vi "RANGE Grab Bank Data.vi"(0 "DAQ Data In in":T4, 1 "Meter Number":T10, 2 "Tot.Flow (Liters) Bank 2":dbl, 3 "Use Mass Flow Unit Converter?":bool, 5 "Meter Select":T3, 7 "Tot.Flow (Liters) Bank 1":dbl, 9 "Meter Select 2":T1, 11 "error in (no error)":errorcluster, 12 "Meter Select 3":T2, 13 "Tot.Flow (Liters) Bank 3":dbl) -> (4 "DAQ Data In out":T4, 15 "error out":errorcluster)   [LabVIEW 2018]
uses:
  Type Definitions/RANGE DAQ Data Four Meters.ctl
  Type Definitions/RANGE DAQ Data.ctl
  Drivers/Omega FMA-1600A Series Gas Flow Meter/Type Definitions/FMA1600A Gas Type.ctl
  Drivers/Omega FMA-1600A Series Gas Flow Meter/Type Definitions/FMA1600A Units String.ctl
  Type Definitions/RANGE GAS Data.ctl
  Type Definitions/RANGE Panel Data.ctl
  Type Definitions/Range Meter Bank.ctl
  Type Definitions/RANGE Meter Selector 1-2.ctl
  Type Definitions/RANGE Meter Selector 5-6.ctl
  Type Definitions/RANGE Meter Selector 3-4.ctl
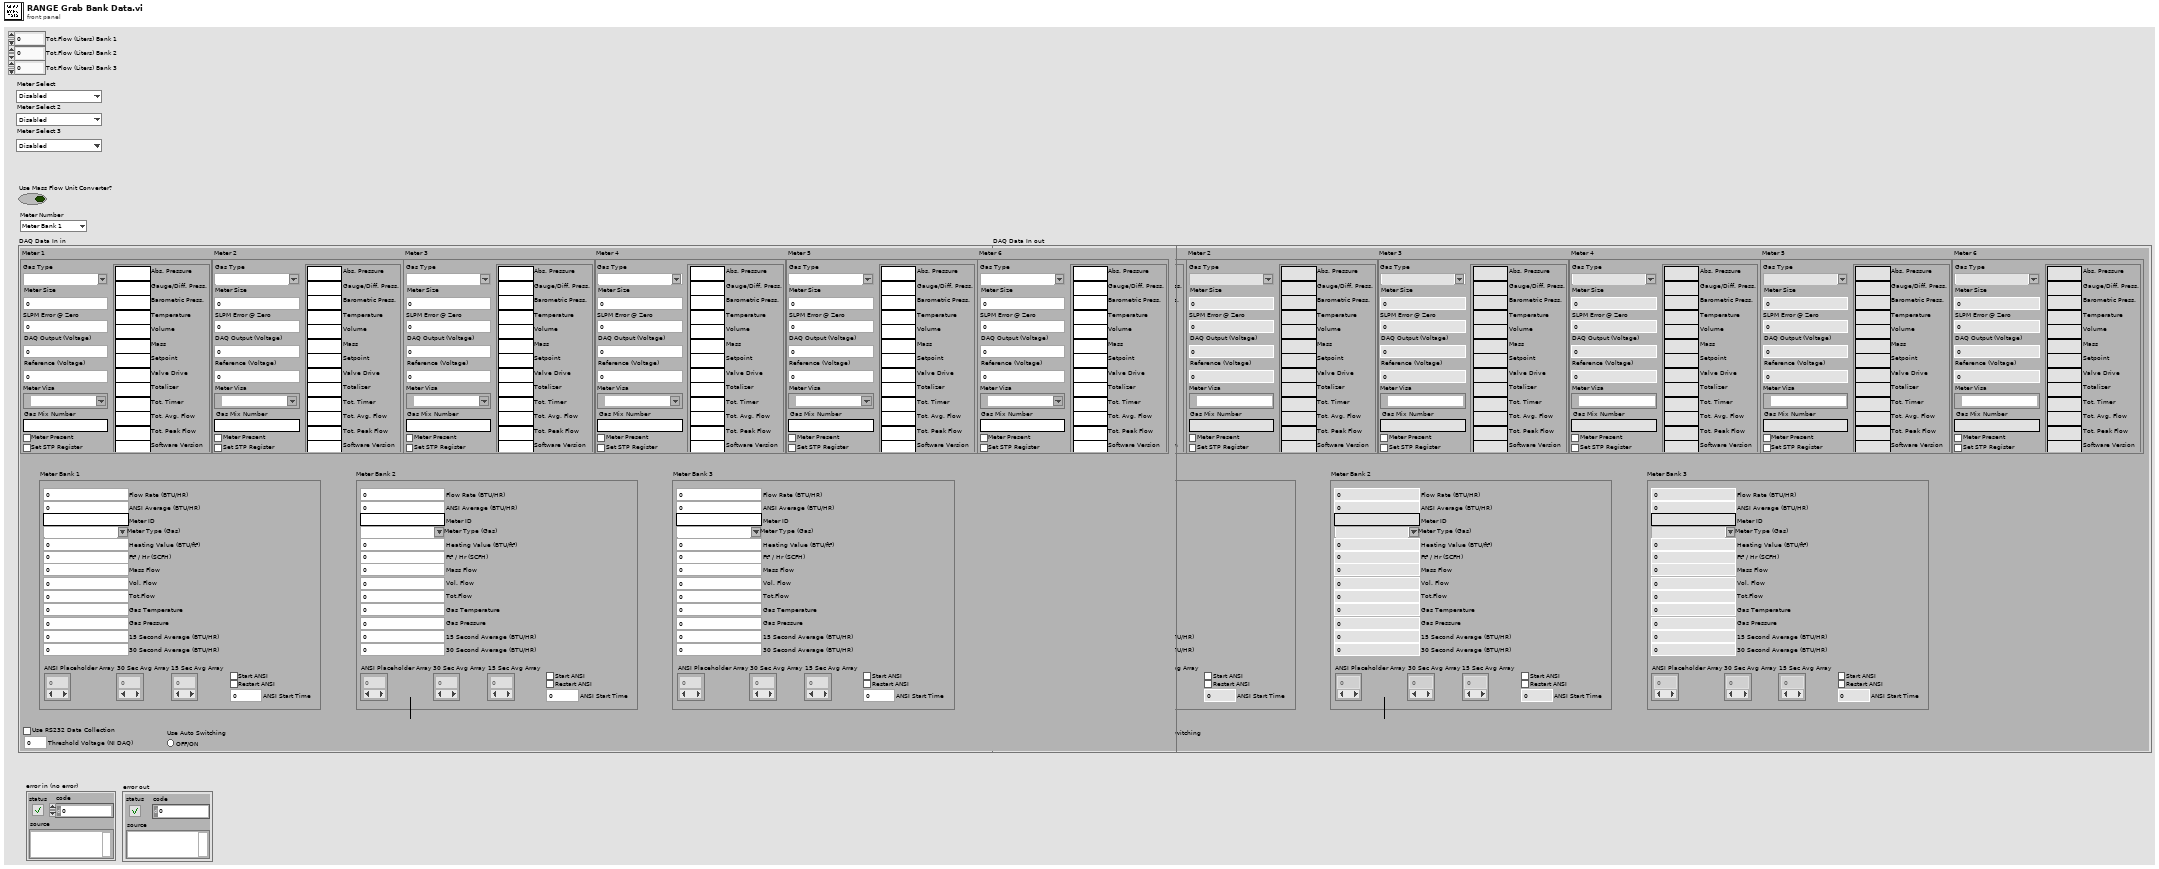
[diagram p1: front panel]
types:
  T1 = typedef "RANGE Meter Selector 3-4.ctl" = enum16{"Disabled", "Meter 3", "Meter 4", "Auto"}
  T2 = typedef "RANGE Meter Selector 5-6.ctl" = enum16{"Disabled", "Meter 5", "Meter 6", "Auto"}
  T3 = typedef "RANGE Meter Selector 1-2.ctl" = enum16{"Disabled", "Meter 1", "Meter 2", "Auto"}
  T4 = typedef "RANGE DAQ Data Four Meters.ctl" = cluster{"Meter 1":T5, "Meter 2":T5, "Meter 3":T5, "Meter 4":T5, "Meter 5":T5, "Meter 6":T5, "Meter Bank 1":T8, "Meter Bank 2":T8, "Meter Bank 3":T8, "Threshold Voltage (NI DAQ)":dbl, "Use RS232 Data Collection":bool, "Use Auto Switching":bool}
  T5 = typedef "RANGE DAQ Data.ctl" = cluster{"Meter Size":dbl, "DAQ Output (Voltage)":dbl, "Reference (Voltage)":dbl, "Meter Present":bool, "Meter Visa":refnum<visa-resource-name>, "Gas Type":T6, "SLPM Error @ Zero":dbl, "Gas Mix Number":string, "Set STP Register":bool, "Measurement Units":T7}
  T6 = typedef "FMA1600A Gas Type.ctl" = string
  T7 = typedef "FMA1600A Units String.ctl" = cluster{"Abs. Pressure":string, "Gauge/Diff. Press.":string, "Barometric Press.":string, "Temperature":string, "Volume":string, "Mass":string, "Setpoint":string, "Valve Drive":string, "Totalizer":string, "Tot. Timer":string, "Tot. Avg. Flow":string, "Tot. Peak Flow":string, "Software Version":string}
  T8 = typedef "RANGE GAS Data.ctl" = cluster{"Flow Rate (BTU/HR)":dbl, "ANSI Placeholder Array":dbl[], "15 Sec Avg Array":dbl[], "30 Sec Avg Array ":dbl[], "ANSI Average (BTU/HR)":dbl, "Panel Data":T9, "Start ANSI":bool, "ANSI Start Time":dbl, "Restart ANSI":bool, "Meter ID":string}
  T9 = typedef "RANGE Panel Data.ctl" = cluster{"Meter Type (Gas)":T6, "Heating Value (BTU/ft³)":dbl, "Ft³ / Hr (SCFH)":dbl, "15 Second Average (BTU/HR)":dbl, "30 Second Average (BTU/HR)":dbl, "Mass Flow":dbl, "Vol. Flow":dbl, "Gas Temperature":dbl, "Gas Pressure":dbl, "Tot.Flow":dbl}
  T10 = typedef "Range Meter Bank.ctl" = enum16{"Meter Bank 1", "Meter Bank 2", "Meter Bank 3"}
  T11 = typedef "FMA1600A Data.ctl" = cluster{"Pressure (PSIA)":dbl, "Temperature (°F)":dbl, "Vol. Flow (LPM)":dbl, "Mass Flow (SLPM)":dbl, "Gas Type":string, "Tot. Flow (Liters)":dbl, "Meter ID":string}
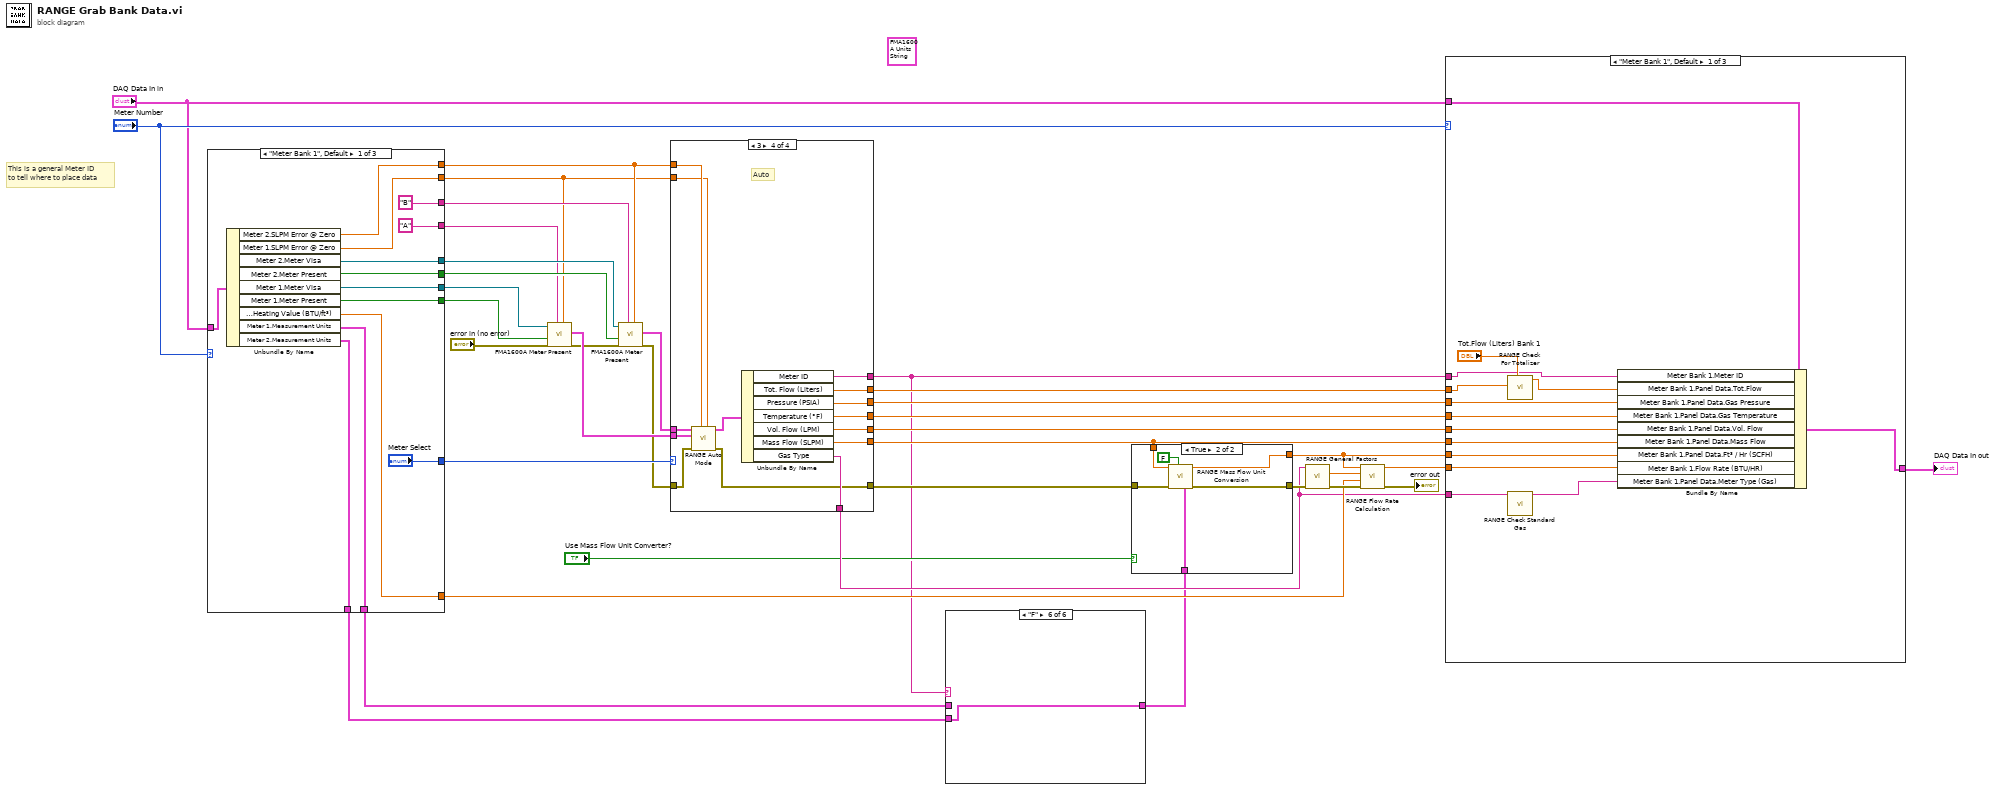
[diagram p0: block diagram]
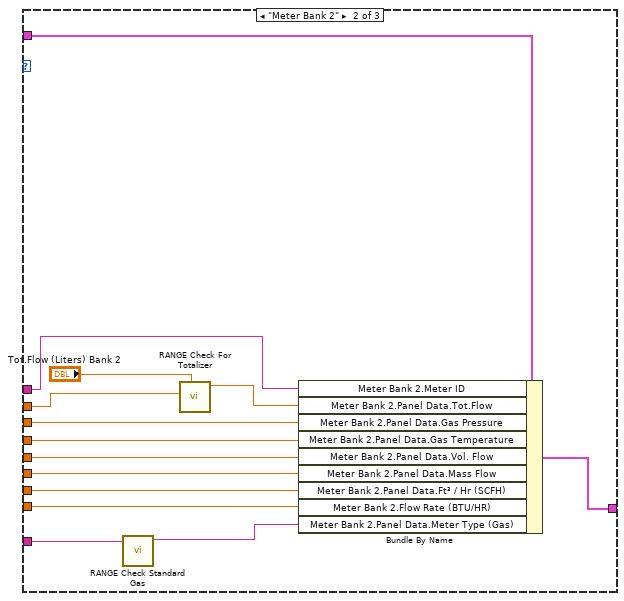
[diagram p8: hidden frame]
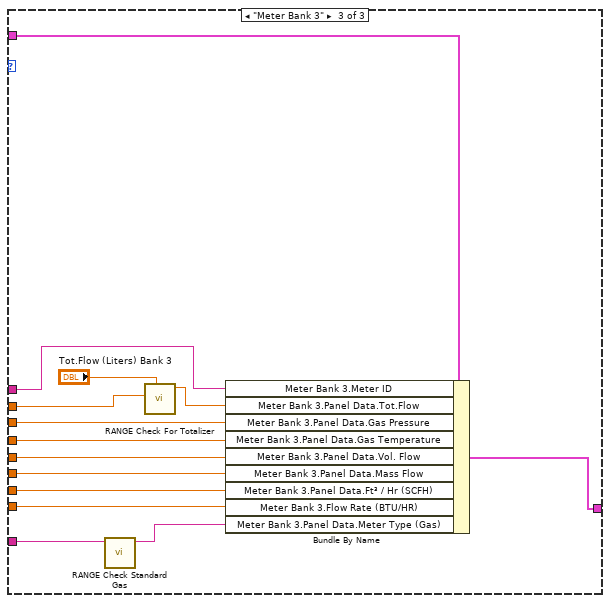
[diagram p9: hidden frame]
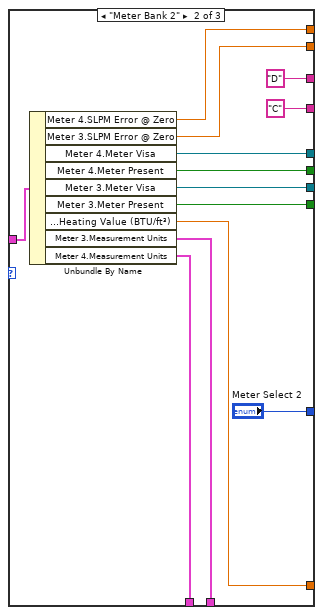
[diagram p10: hidden frame]
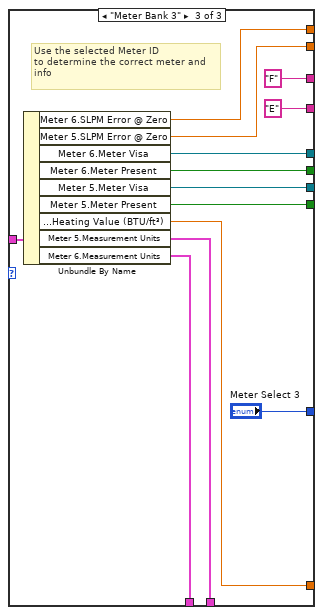
[diagram p11: hidden frame]
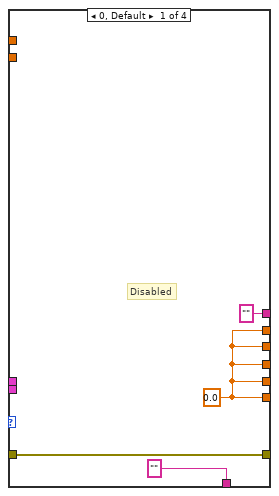
[diagram p12: hidden frame]
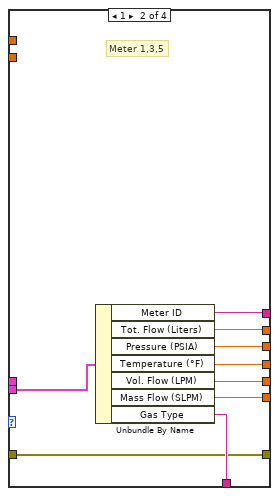
[diagram p13: hidden frame]
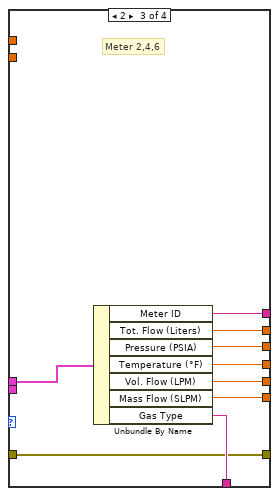
[diagram p14: hidden frame]
diagram:
  (unwired) T7 {"Abs. Pressure"="", "Gauge/Diff. Press."="", "Barometric Press."="", "Temperature"="", "Volume"="", "Mass"="", "Setpoint"="", "Valve Drive"="", "Totalizer"="", "Tot. Timer"="", "Tot. Avg. Flow"="", "Tot. Peak Flow"="", "Software Version"=""} ("Measurement Units")
  # "This is a general Meter ID\nto tell where to place data"
  n1 = case shown="\"Meter Bank 1\", Default" "Meter Number" {
    tunnel: ["A" ("Unit ID") "C" ("Unit ID") "E" ("Unit ID")] -> w22
    tunnel: [w48 w58 w71] -> w5
    tunnel: ["B" ("Unit ID") "D" ("Unit ID") "F" ("Unit ID")] -> w21
    tunnel: "DAQ Data In in" -> [w46 w60 w73]
    tunnel: ["Meter Select" "Meter Select 2" "Meter Select 3"] -> w34
    tunnel: [w45 w59 w72] -> w25
    tunnel: [w44 w57 w70] -> w27
    tunnel: [w43 w56 w69] -> w24
    tunnel: [w42 w55 w67] -> w7
    tunnel: [w41 w54 w68] -> w6
    tunnel: [w40 w53 w66] -> w13
    tunnel: [w38 w50 w63] -> w2
    tunnel: [w37 w51 w64] -> w3
    frame "Meter Bank 1", Default {
      n2 = Unbundle By Name(w46) -> ("Meter 2.SLPM Error @ Zero"=w42:dbl, "Meter 1.SLPM Error @ Zero"=w41:dbl, "Meter 2.Meter Visa"=w45:refnum<visa-resource-name>, "Meter 2.Meter Present"=w43:bool, "Meter 1.Meter Visa"=w48:refnum<visa-resource-name>, "Meter 1.Meter Present"=w44:bool, "Meter Bank 1.Panel Data.Heating Value (BTU/ft³)"=w40:dbl, "Meter 1.Measurement Units"=w37:T7, "Meter 2.Measurement Units"=w38:T7)
    }
    frame "Meter Bank 2" {
      n3 = Unbundle By Name(w60) -> ("Meter 4.SLPM Error @ Zero"=w55:dbl, "Meter 3.SLPM Error @ Zero"=w54:dbl, "Meter 4.Meter Visa"=w59:refnum<visa-resource-name>, "Meter 4.Meter Present"=w56:bool, "Meter 3.Meter Visa"=w58:refnum<visa-resource-name>, "Meter 3.Meter Present"=w57:bool, "Meter Bank 2.Panel Data.Heating Value (BTU/ft³)"=w53:dbl, "Meter 3.Measurement Units"=w51:T7, "Meter 4.Measurement Units"=w50:T7)
    }
    frame "Meter Bank 3" {
      # "Use the selected Meter ID\nto determine the correct meter and\ninfo"
      n4 = Unbundle By Name(w73) -> ("Meter 6.SLPM Error @ Zero"=w67:dbl, "Meter 5.SLPM Error @ Zero"=w68:dbl, "Meter 6.Meter Visa"=w72:refnum<visa-resource-name>, "Meter 6.Meter Present"=w69:bool, "Meter 5.Meter Visa"=w71:refnum<visa-resource-name>, "Meter 5.Meter Present"=w70:bool, "Meter Bank 3.Panel Data.Heating Value (BTU/ft³)"=w66:dbl, "Meter 5.Measurement Units"=w64:T7, "Meter 6.Measurement Units"=w63:T7)
    }
  }
  n5 = call "FMA1600A Meter Present.vi"("SLPM Error @ Zero"=w6, "Unit ID"=w22, "error in (no error)"="error in (no error)", "Meter Present"=w27, "VISA Refnum in"=w5) -> ("error out"=w26:errorcluster, "FMA1600A Gas Data"=w30:T11)  [unwired: 5 in]
  n6 = call "FMA1600A Meter Present.vi"("SLPM Error @ Zero"=w7, "Unit ID"=w21, "error in (no error)"=w26, "Meter Present"=w24, "VISA Refnum in"=w25) -> ("error out"=w9:errorcluster, "FMA1600A Gas Data"=w23:T11)  [unwired: 5 in]
  n7 = case shown="3" w34 {
    tunnel: w30 -> [_ w88 _ w111]
    tunnel: [w78 w87 w96 w107] -> w31
    tunnel: [w78 w86 w95 w106] -> w32
    tunnel: [w78 w85 w94 w105] -> w33
    tunnel: [w78 w84 w93 w104] -> w20
    tunnel: w23 -> [_ _ w97 w110]
    tunnel: ["" ("Gas Type") w83 w92 w103] -> w12
    tunnel: [w78 w82 w91 w108] -> w10
    tunnel: w9 -> [w77 w81 w90 w102]
    tunnel: [w77 w81 w90 w101] -> w8
    tunnel: w7 -> [_ _ _ w100]
    tunnel: w6 -> [_ _ _ w99]
    tunnel: ["" ("Meter ID") w80 w89 w98] -> w4
    frame 0, Default {
      w78 = 0.0 ("Pressure (PSIA)")
      # "Disabled"
    }
    frame 1 {
      # "Meter 1,3,5"
      n8 = Unbundle By Name(w88) -> ("Meter ID"=w80:string, "Tot. Flow (Liters)"=w82:dbl, "Pressure (PSIA)"=w87:dbl, "Temperature (°F)"=w86:dbl, "Vol. Flow (LPM)"=w85:dbl, "Mass Flow (SLPM)"=w84:dbl, "Gas Type"=w83:string)
    }
    frame 2 {
      # "Meter 2,4,6"
      n9 = Unbundle By Name(w97) -> ("Meter ID"=w89:string, "Tot. Flow (Liters)"=w91:dbl, "Pressure (PSIA)"=w96:dbl, "Temperature (°F)"=w95:dbl, "Vol. Flow (LPM)"=w94:dbl, "Mass Flow (SLPM)"=w93:dbl, "Gas Type"=w92:string)
    }
    frame 3 {
      # "Auto"
      n10 = call "RANGE Auto Mode.vi"("SLPM Error @ Zero (2,4,6)"=w99, "SLPM Error @ Zero (1,3,5)"=w100, "Error In"=w102, "Meter 1,3,5"=w111, "Meter 2,4,6"=w110) -> ("Error Out"=w101:errorcluster, "Meter Auto"=w109:T11)  [unwired: 4 in, 1 out]
      n11 = Unbundle By Name(w109) -> ("Meter ID"=w98:string, "Tot. Flow (Liters)"=w108:dbl, "Pressure (PSIA)"=w107:dbl, "Temperature (°F)"=w106:dbl, "Vol. Flow (LPM)"=w105:dbl, "Mass Flow (SLPM)"=w104:dbl, "Gas Type"=w103:string)
    }
  }
  n12 = case shown="\"F\"" w4 {
    tunnel: w3 -> [w112 _ w114 _ w116 _]
    tunnel: w2 -> [_ w113 _ w115 _ w117]
    tunnel: [w112 w113 w114 w115 w116 w117] -> w1
    frame "A", Default {
    }
    frame "B" {
    }
    frame "C" {
    }
    frame "D" {
    }
    frame "E" {
    }
    frame "F" {
    }
  }
  n13 = case shown="True" "Use Mass Flow Unit Converter?" {
    tunnel: w20 -> [w118 w125]
    tunnel: [w119 w123] -> w17
    tunnel: [w118 w122] -> w15
    tunnel: w8 -> [w119 w121]
    tunnel: w1 -> [_ w120]
    frame False {
    }
    frame True {
      n14 = call "RANGE Mass Flow Unit Conversion.vi"("Meter Units Out"=w120, "Ft³/HR -SLPM (T)"=FALSE, "Error In"=w121, "Input Mass Flow Rate"=w125) -> ("Error Out"=w123:errorcluster, "Output Mass Flow Rate"=w122:dbl)  [unwired: 6 in]
    }
  }
  n15 = call "RANGE General Factors.vi"("Error In"=w17, "Gas Type String"=w12) -> ("Error Out"=w18:errorcluster, "Flow Rate Factor"=w19:dbl)  [unwired: 8 in]
  n16 = call "RANGE Flow Rate Calculation.vi"("Error In"=w18, "Heating Value (BTU/ft³)"=w13, "Flow Rate Factor"=w19, "Ft³/HR"=w15) -> ("Error Out"=→"error out":errorcluster, "Flow Rate (BTU/Hr)"=w16:dbl)  [unwired: 6 in]
  n17 = case shown="\"Meter Bank 1\", Default" "Meter Number" {
    tunnel: "DAQ Data In in" -> [w139 w153 w167]
    tunnel: w31 -> [w138 w150 w166]
    tunnel: w32 -> [w137 w149 w165]
    tunnel: w33 -> [w136 w148 w164]
    tunnel: w20 -> [w135 w147 w163]
    tunnel: [w134 w152 w162] -> w36
    tunnel: w15 -> [w132 w146 w161]
    tunnel: w16 -> [w133 w145 w160]
    tunnel: w12 -> [w131 w144 w159]
    tunnel: w10 -> [w129 w143 w157]
    tunnel: w4 -> [w126 w140 w154]
    frame "Meter Bank 1", Default {
      n18 = call "RANGE Check For Totalizer.vi"("Calculated Totalizer"="Tot.Flow (Liters) Bank 1", "Meter Totalizer"=w129) -> ("Tot. Flow (Liters) out"=w128:dbl)  [unwired: 9 in]
      n19 = call "RANGE Check Standard Gas.vi"("Gas Type"=w131) -> ("Gas Type"=w130:string)  [unwired: 9 in, 1 out]
      n20 = Bundle By Name(cluster=w139, "Meter Bank 1.Meter ID"=w126, "Meter Bank 1.Panel Data.Tot.Flow"=w128, "Meter Bank 1.Panel Data.Gas Pressure"=w138, "Meter Bank 1.Panel Data.Gas Temperature"=w137, "Meter Bank 1.Panel Data.Vol. Flow"=w136, "Meter Bank 1.Panel Data.Mass Flow"=w135, "Meter Bank 1.Panel Data.Ft³ / Hr (SCFH)"=w132, "Meter Bank 1.Flow Rate (BTU/HR)"=w133, "Meter Bank 1.Panel Data.Meter Type (Gas)"=w130) -> (w134:T4)
    }
    frame "Meter Bank 2" {
      n21 = call "RANGE Check Standard Gas.vi"("Gas Type"=w144) -> ("Gas Type"=w151:string)  [unwired: 9 in, 1 out]
      n22 = call "RANGE Check For Totalizer.vi"("Calculated Totalizer"="Tot.Flow (Liters) Bank 2", "Meter Totalizer"=w143) -> ("Tot. Flow (Liters) out"=w142:dbl)  [unwired: 9 in]
      n23 = Bundle By Name(cluster=w153, "Meter Bank 2.Meter ID"=w140, "Meter Bank 2.Panel Data.Tot.Flow"=w142, "Meter Bank 2.Panel Data.Gas Pressure"=w150, "Meter Bank 2.Panel Data.Gas Temperature"=w149, "Meter Bank 2.Panel Data.Vol. Flow"=w148, "Meter Bank 2.Panel Data.Mass Flow"=w147, "Meter Bank 2.Panel Data.Ft³ / Hr (SCFH)"=w146, "Meter Bank 2.Flow Rate (BTU/HR)"=w145, "Meter Bank 2.Panel Data.Meter Type (Gas)"=w151) -> (w152:T4)
    }
    frame "Meter Bank 3" {
      n24 = call "RANGE Check Standard Gas.vi"("Gas Type"=w159) -> ("Gas Type"=w158:string)  [unwired: 9 in, 1 out]
      n25 = call "RANGE Check For Totalizer.vi"("Calculated Totalizer"="Tot.Flow (Liters) Bank 3", "Meter Totalizer"=w157) -> ("Tot. Flow (Liters) out"=w156:dbl)  [unwired: 9 in]
      n26 = Bundle By Name(cluster=w167, "Meter Bank 3.Meter ID"=w154, "Meter Bank 3.Panel Data.Tot.Flow"=w156, "Meter Bank 3.Panel Data.Gas Pressure"=w166, "Meter Bank 3.Panel Data.Gas Temperature"=w165, "Meter Bank 3.Panel Data.Vol. Flow"=w164, "Meter Bank 3.Panel Data.Mass Flow"=w163, "Meter Bank 3.Panel Data.Ft³ / Hr (SCFH)"=w161, "Meter Bank 3.Flow Rate (BTU/HR)"=w160, "Meter Bank 3.Panel Data.Meter Type (Gas)"=w158) -> (w162:T4)
    }
  }
  "DAQ Data In out" <- w36
